vi "Load Unload Application.vi"(0 "VISA resource name":refnum<visa-resource-name>, 5 "Application Operation  (0:Load)":i32(ring) items=["Load", "Unload"], 7 "Application Name (1:Spectrum Analyzer)":i32(ring)=1 items=["Signal Analyzer", "Spectrum Analyzer", "Phase Noise", "Config", "Signal Generator", "BER Test", "WiMAX", "W-CDMA/HSPA Downlink", "W-CDMA/HSPA Uplink", "GSM", "ETC/DSRC", "TD-SCDMA", "XG-PHS", "Vector Modulation Analysis", "3GLTE Downlink", "3GLTE Uplink", "LTE-TDD Downlink", "CDMA2000", "EVDO", "W-CDMA BS", "W-CDMA RNC Simulator Control", "MediaFLO", "ISDB-Tmm", "UMTS Measurement Software", "Digital I/F Control Software", "PA Measurement", "Power Meter"], 11 "error in (no error)":errorcluster) -> (4 "VISA resource name out":refnum<visa-resource-name>, 15 "error out":errorcluster)   [LabVIEW 2020, in "Anritsu Signal Analyzer Series.lvlib"]
doc: "Loads or Unloads an application."
uses:
  Anritsu Signal Analyzer Series.lvlib
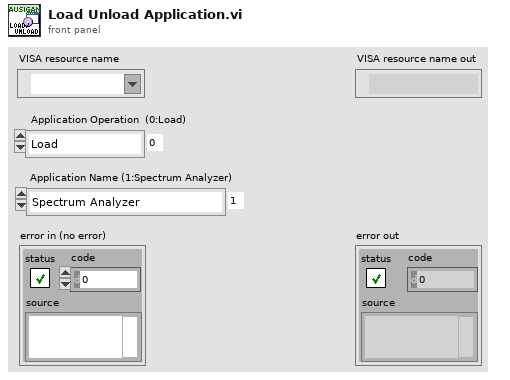
[diagram p1: front panel]
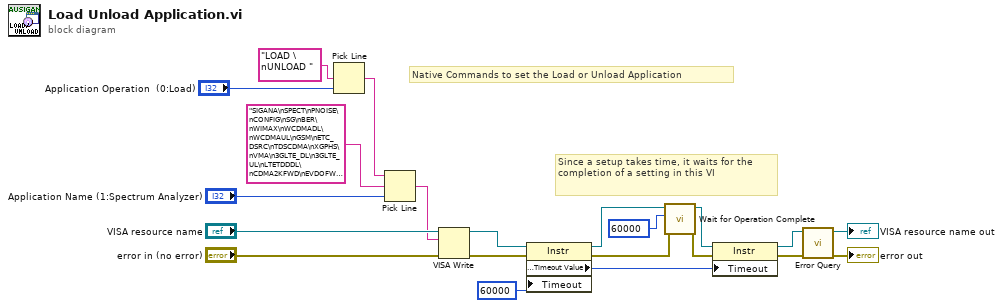
[diagram p0: block diagram]
diagram:
  # "Since a setup takes time, it waits for the completion of a setting in this VI"
  # "Native Commands to set the Load or Unload Application"
  n1 = Pick Line(multi-line string="LOAD \nUNLOAD " ("_Command"), line index="Application Operation  (0:Load)") -> (output string=w13:string)  [unwired: 1 in]
  n2 = Pick Line(string ("")=w13, multi-line string="SIGANA\nSPECT\nPNOISE\nCONFIG\nSG\nBER\nWIMAX\nWCDMADL\nWCDMAUL\nGSM\nETC_DSRC\nTDSCDMA\nXGPHS\nVMA\n3GLTE_DL\n3GLTE_UL\nLTETDDDL\nCDMA2KFWD\nEVDOFWD\nWCDMA_BS\nRNC\nMEDIAFLO\nISDBTMM\nUMTS\nBBIF\nPA\nPMET" ("文字列"), line index="Application Name (1:Spectrum Analyzer)") -> (output string=w14:string)
  n3 = VISA Write(VISA resource name="VISA resource name", write buffer=w14, error in (no error)="error in (no error)") -> (VISA resource name out=w10:refnum<visa-resource-name>, error out=w9:errorcluster)  [unwired: 1 out]
  n4 = property class="Instr"(reference=w10, error in=w9, "Timeout"=u32 60000 ("General Settings:Timeout Value")) -> (reference out=w7:refnum<visa-resource-name>, error out=w8:errorcluster, "General Settings:Timeout Value"=w1:u32)
  n5 = call "Wait for Operation Complete.vi"("error in (no error)"=w8, "Maximum Time (10000mSec)"=60000 ("Maximum Time (60000mSec)"), "VISA resource name"=w7) -> ("error out"=w2:errorcluster, "VISA resource name out"=w5:refnum<visa-resource-name>)  [unwired: 7 in]
  n6 = property class="Instr"(reference=w5, error in=w2, "Timeout"=w1) -> (reference out=w4:refnum<visa-resource-name>, error out=w3:errorcluster)
  n7 = call "Error Query.vi"("error in (no error)"=w3, "VISA resource name"=w4) -> ("error out"=→"error out":errorcluster, "VISA resource name out"=→"VISA resource name out":refnum<visa-resource-name>)  [unwired: 6 in, 2 out]
